vi "Sleep H2 Sensor Loop.vi"(8 "error in":errorcluster) -> (0 "error out":errorcluster)   [LabVIEW 2024, in "Anode.lvlib"]
doc: "Sleeps the H2 Sensor CAN bus Helper Loop\n\n_____\nCreated using DQMH Framework: Event Scripter 7.1.1.1528."
uses:
  Anode.lvlib
  Sleep H2 Sensor Loop Argument--cluster.ctl
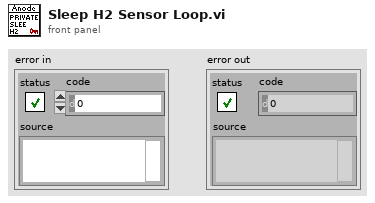
[diagram p1: front panel]
types:
  T1 = typedef "Anode.lvlib/Sleep H2 Sensor Loop Argument--cluster.ctl" = cluster{"Boolean":bool}
  T2 = typedef "Anode.lvlib/Request Events--cluster.ctl" = cluster{"Stop Module":refnum<user-event>, "Show Panel":refnum<user-event>, "Hide Panel":refnum<user-event>, "Get Module Execution Status":refnum<user-event>, "Show Diagram":refnum<user-event>, "Change Panel":refnum<user-event>, "Set Anode Inlet Pressure SP":refnum<user-event>, "Initialise Pressure Regulator Interface":refnum<user-event>, "Start Polling Pressure Regulator Status":refnum<user-event>, "Stop Polling Pressure Regulator Status":refnum<user-event>, "Read Pressure Regulator Status":refnum<user-event>, "Set Pressure Regulator Control Function":refnum<user-event>, "Set Anode Inlet Flow SP":refnum<user-event>, "Set Anode Inlet Valve State":refnum<user-event>, "Private":cluster{"Wake Connection Helper Loop":refnum<user-event>}, "Set Anode Gas Supply Valve":refnum<user-event>, "Set Purge Valve":refnum<user-event>, "Set Purge Strategy":refnum<user-event>, "Private.Wake Purge Strategy Helper Loop":refnum<user-event>, "Private.Update Purge Strategy Settings":refnum<user-event>, "Wake Purge Helper Loop":refnum<user-event>, "Wake Recirculation Pump Helper Loop":refnum<user-event>, "Sleep Recirculation Pump Helper Loop":refnum<user-event>, "Set Pump Speed SP":refnum<user-event>, "Set Pump Enable State":refnum<user-event>, "Set Pump Speed Control Mode":refnum<user-event>, "Private.Update Purge Strategy Helper Loop":refnum<user-event>, "Force Purge":refnum<user-event>, "Reset Counter":refnum<user-event>, "Private.Wake H2 Sensor Loop":refnum<user-event>, "Private.Sleep H2 Sensor Loop":refnum<user-event>, "Start H2 Sensor Measurement":refnum<user-event>, "Stop H2 Sensor Measurement":refnum<user-event>}
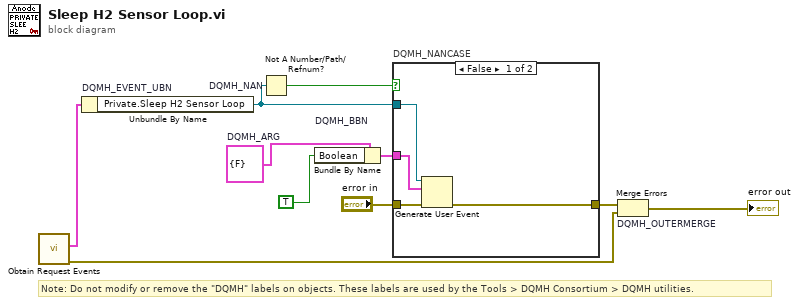
[diagram p0: block diagram]
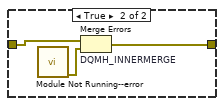
[diagram p2: hidden frame]
diagram:
  w4 = T1 {"Boolean"=FALSE}  # DQMH_ARG
  # "Note: Do not modify or remove the \"DQMH\" labels on objects. These labels are used by the Tools > DQMH Consortium > DQMH utilities."
  n1 = call "Obtain Request Events.vi"() -> ("error out"=w2:errorcluster, "Anode Request Events"=w1:T2)  [unwired: 10 in]
  n2 = Unbundle By Name "DQMH_EVENT_UBN"(w1) -> ("Private.Sleep H2 Sensor Loop"=w6:refnum<user-event>)
  n3 = Not A Number/Path/Refnum? "DQMH_NAN"(number/path/refnum=w6) -> (NaN/Path/Refnum?=w7:bool)
  n4 = Bundle By Name "DQMH_BBN"(cluster=w4, "Boolean"=TRUE) -> (w8:T1)
  n5 = case "DQMH_NANCASE" shown="False" w7 {
    tunnel: "error in" -> [w14 w17]
    tunnel: [w13 w16] -> w5
    tunnel: w6 -> [w12 _]
    tunnel: w8 -> [w11 _]
    frame False {
      n6 = Generate User Event(user event=w12, event data cluster=w11, error in=w14) -> (error out=w13:errorcluster)  [unwired: 1 in, 1 out]
    }
    frame True {
      n7 = call "Module Not Running--error.vi"() -> ("error out"=w15:errorcluster)  [unwired: 11 in]
      n8 = Merge Errors "DQMH_INNERMERGE"(w17, w15) -> (w16:errorcluster)
    }
  }
  n9 = Merge Errors "DQMH_OUTERMERGE"(w5, w2) -> (→"error out":errorcluster)
